vi "Read XML.vi"() -> (0 "error out":errorcluster caption="错误输出", 3 "值":T1)   [LabVIEW 2016]
uses:
  <vilib>/Utility/xml.llb/Read From XML File(string).vi
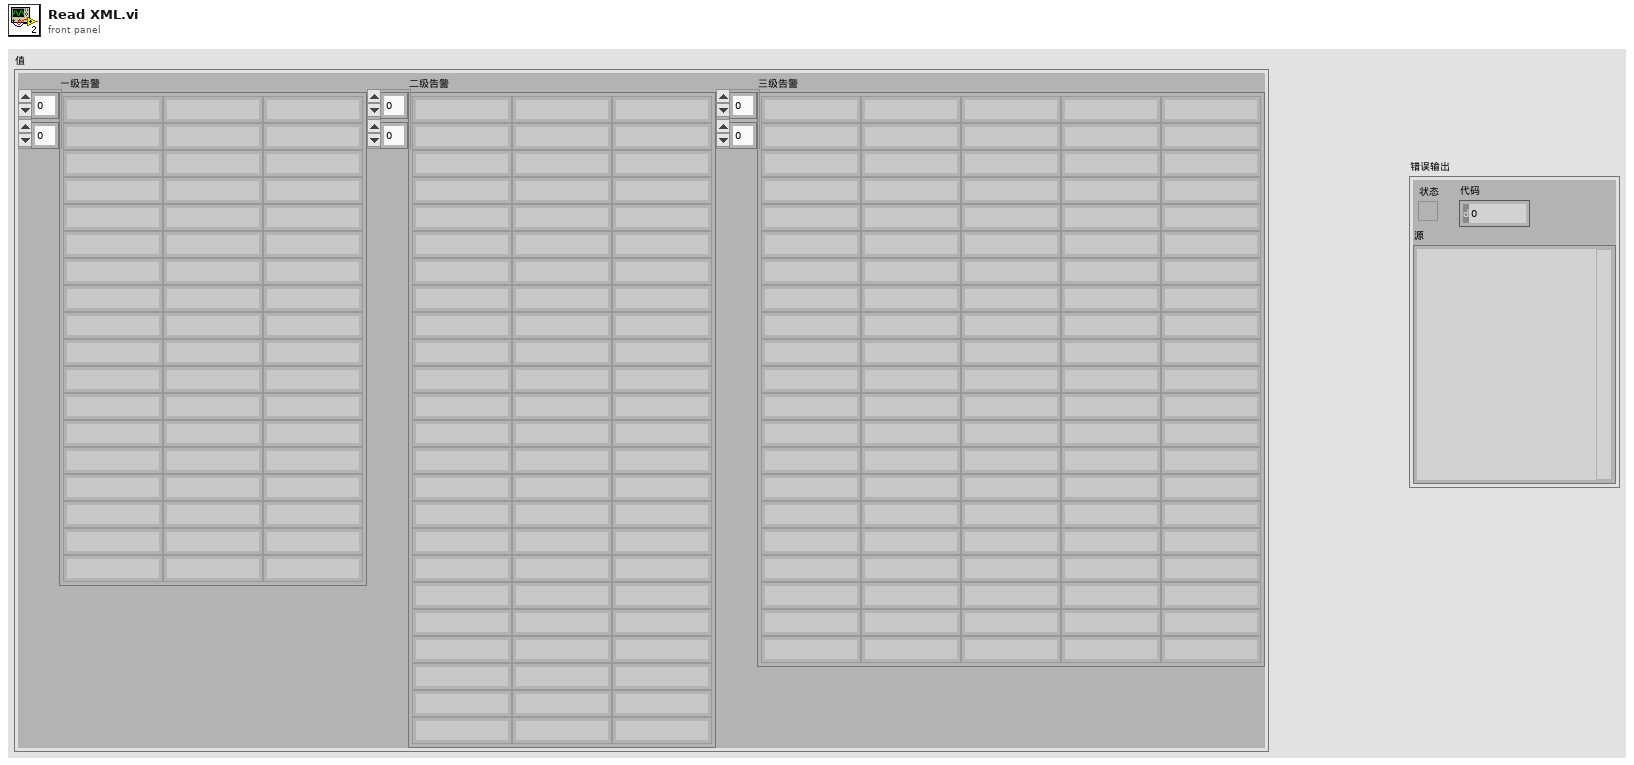
[diagram p1: front panel]
types:
  T1 = cluster{"一级告警":string[][], "二级告警":string[][], "三级告警":string[][]}
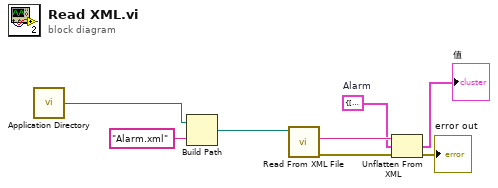
[diagram p0: block diagram]
diagram:
  w4 = T1 {"一级告警"=[], "二级告警"=[], "三级告警"=[]}  # Alarm
  n1 = call <vilib>:"Application Directory.vi"() -> ("Application Directory"=w2:path)
  n2 = Build Path(base path=w2, name or relative path="Alarm.xml" ("名称或相对路径")) -> (appended path=w5:path)
  n3 = call-poly <vilib>:"Read From XML File.vi"("XML File Path"=w5) -> ("error out"=w1:errorcluster, "XML Elements"=w8:string)  [unwired: 8 in, 1 out]
  n4 = Unflatten From XML(xml string=w8, type=w4, error in (no error)=w1) -> (value=→"值":T1, error out=→"error out":errorcluster)
